vi "REWORK_create_menu_bar.vi"(8 "error_in":errorcluster, 11 "menu_bar_refnum":refnum<k9>) -> (0 "error_out":errorcluster)   [LabVIEW 2019]
doc: "This VI creates menu bar for main GUI window, populates menus with appropriate items and creates keyboard shortcuts. To work properly it needs menu.rtm file, which contains base for custom menu bar creation. \nLabVIEW can not create custom menu from scratch, only by editing existing custom menu created with editor (Edit -> Run-Time Menu...). File menu.rtm contains one element, 'placeholder', which is deleted \n(from menu, not from file) at the beginning of menu creation, and then whole menu is created programatically. This way whole menu can be edited without need to change menu.rtm file.\n\nLink refnum obtained from Current VI's Menubar.vi to menu_bar_refnum input of this vi."
uses:
  _misc/AULocalize/SubVIs/Get Localized Phrase Compact Interface 1D.vi
  _misc/AULocalize/SubVIs/Get Localized Phrase Compact Interface 0D.vi
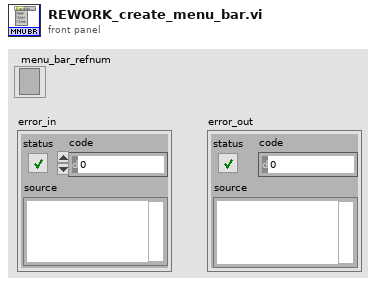
[diagram p1: front panel]
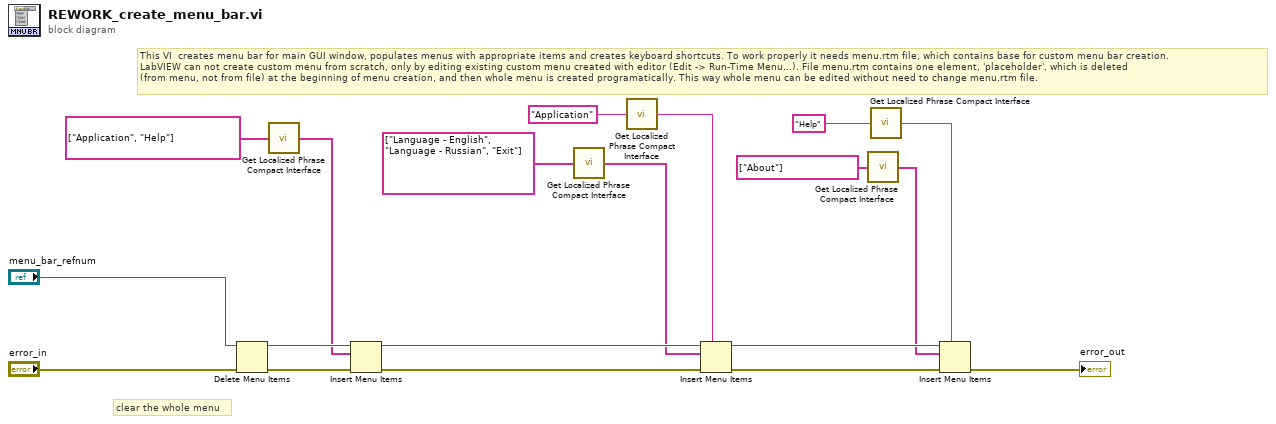
[diagram p0: block diagram]
diagram:
  # "clear the whole menu"
  # "This VI  creates menu bar for main GUI window, populates menus with appropriate items and creates keyboard shortcuts. To work properly it needs menu.rtm file, which contains base for custom menu bar creation. \nLabVIEW can not create custom menu from scratch, only by editing existing custom menu created with editor (Edit -> Run-Time Menu...). File menu.rtm contains one element, 'placeholder', which is deleted \n(from menu, not from file) at the beginning of menu creation, and then whole menu is created programatically. This way whole menu can be edited without need to change menu.rtm file."
  n1 = Delete Menu Items(6:"error_in", 9:"menu_bar_refnum") -> (0:w16:errorcluster, 3:w17:refnum<k9>)  [unwired: 2 in]
  n2 = call-poly "Get Localized Phrase Compact Interface.vi"("Key"=string[] ["Application", "Help"] ("item names")) -> ("Translated Phrase"=w10:string[])
  n3 = Insert Menu Items(6:w16, 8:w10, 9:w17) -> (0:w15:errorcluster, 3:w14:refnum<k9>)  [unwired: 3 in, 1 out]
  n4 = call-poly "Get Localized Phrase Compact Interface.vi"("Key"=string[] ["Language - English", "Language - Russian", "Exit"] ("item names")) -> ("Translated Phrase"=w8:string[])
  n5 = call-poly "Get Localized Phrase Compact Interface.vi"("Key"="Application" ("menu tag")) -> ("Translated Phrase"=w6:string)
  n6 = Insert Menu Items(5:w6, 6:w15, 8:w8, 9:w14) -> (0:w13:errorcluster, 3:w12:refnum<k9>)  [unwired: 2 in, 1 out]
  n7 = call-poly "Get Localized Phrase Compact Interface.vi"("Key"=string[] ["About"] ("item names")) -> ("Translated Phrase"=w4:string[])
  n8 = call-poly "Get Localized Phrase Compact Interface.vi"("Key"="Help" ("menu tag")) -> ("Translated Phrase"=w2:string)
  n9 = Insert Menu Items(5:w2, 6:w13, 8:w4, 9:w12) -> (0:→"error_out":errorcluster)  [unwired: 2 in, 2 out]
